vi "Set Frequency Reference.vi"(8 "error in (no error)":errorcluster, 11 "VISA resource name":refnum<visa-resource-name>) -> (0 "error out":errorcluster, 3 "VISA resource name out":refnum<visa-resource-name>)   [LabVIEW 2012, in "Agilent PSG MXG Series.lvlib"]
doc: "Sets the current output frequency, along with any offset, as a 0 hertz reference value.\n\n<B>Notes:</B>\n(1) This VI is valid only in E8257D, E8267D, N5161A, N5162A, N5181A, N5182A, N5183A, N5171B, N5172B, N5181B, N5182B."
uses:
  <instrlib>/Agilent PSG MXG Series/Agilent PSG MXG Series.lvlib
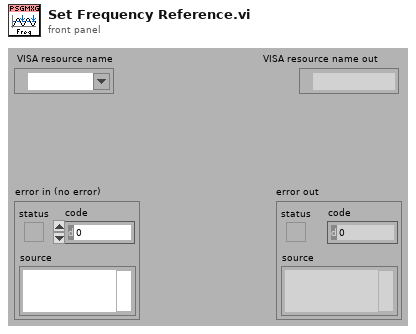
[diagram p1: front panel]
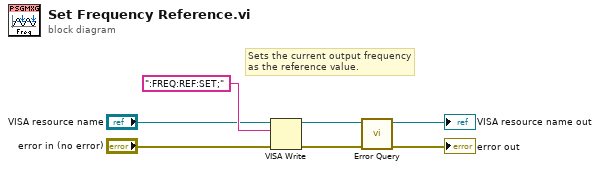
[diagram p0: block diagram]
diagram:
  # "Sets the current output frequency\nas the reference value."
  n1 = VISA Write(VISA resource name="VISA resource name", write buffer=":FREQ:REF:SET;" ("t"), error in (no error)="error in (no error)") -> (VISA resource name out=w7:refnum<visa-resource-name>, error out=w6:errorcluster)  [unwired: 1 out]
  n2 = call <instrlib>:"Error Query.vi"("error in (no error)"=w6, "VISA resource name"=w7) -> ("error out"=→"error out":errorcluster, "VISA resource name out"=→"VISA resource name out":refnum<visa-resource-name>)  [unwired: 8 out]
